vi "Communication - Respond Checker.vi"(11 "Read Data":u8[](array[numeric])) -> (3 "Success":bool)   [LabVIEW 2019]
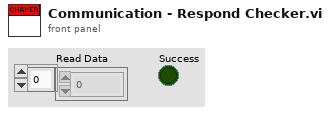
[diagram p1: front panel]
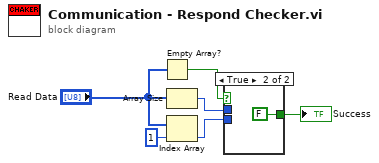
[diagram p0: block diagram]
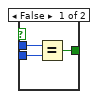
[diagram p2: hidden frame]
diagram:
  n1 = Empty Array?(array="Read Data") -> (empty?=w1:bool)
  n2 = Array Size(array="Read Data") -> (size(s)=w4:i32)
  n3 = Index Array(array="Read Data", index=1) -> (element=w5:u8)
  n4 = case shown="True" w1 {
    tunnel: [w9 FALSE] -> w6
    tunnel: w5 -> [w8 _]
    tunnel: w4 -> [w7 _]
    frame False {
      n5 = Equal?(x=w7, y=w8) -> (x = y?=w9:bool)
    }
    frame True {
    }
  }
  "Success" <- w6
